vi "Check Slave Name.vi"(8 "error in (no error)":errorcluster, 9 "Prepend in":bool, 10 "Slave Name In":string, 11 "Item Ref in":T1 format="%.0x") -> (0 "error out":errorcluster, 1 "Prepend out":bool, 2 "Available?":bool, 3 "Item Ref out":T1 format="%.0x", 4 "Slave Name":string)   [LabVIEW 2020, in "SEECD System Explorer.lvlib"]
uses:
  SEECD System Explorer.lvlib
  <vilib>/NI VeriStand/Custom Device API/Custom Device API.lvlib
  <vilib>/NI VeriStand/Custom Device API/Custom Device Item Ref.ctl
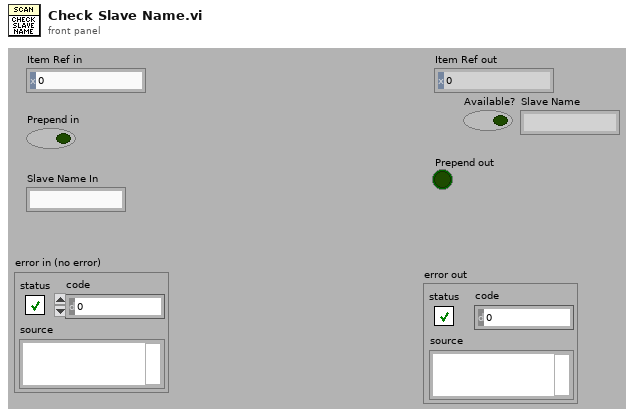
[diagram p1: front panel]
types:
  T1 = typedef "Custom Device API.lvlib/Custom Device Item Ref.ctl" = u64
  T2 = typedef "Custom Device API.lvlib/Custom Device Item Info.ctl" = cluster{"Name":string, "Is Channel":bool, "GUID":string, "Is Waveform":bool}
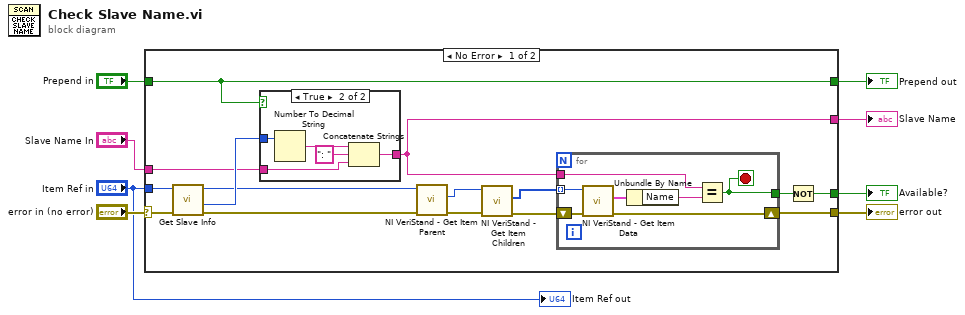
[diagram p0: block diagram]
diagram:
  n1 = case shown="No Error" "error in (no error)" {
    selector: "error in (no error)" -> [w15 w38]
    tunnel: [w20 w38] -> w7
    tunnel: "Item Ref in" -> [w16 _]
    tunnel: "Prepend in" -> [w14 w37]
    tunnel: [w14 w37] -> w5
    tunnel: [w19 _] -> w4
    tunnel: [w10 _] -> w2
    tunnel: "Slave Name In" -> [w9 _]
    frame No Error {
      n2 = call "Get Slave Info.vi"("error in (no error)"=w15, "Item Ref in"=w16) -> ("error out"=w11:errorcluster, "Slave #"=w13:u16, "Item Ref out"=w12:T1)  [unwired: 4 in, 3 out]
      n3 = case shown="True" w14 {
        tunnel: [w24 w29] -> w10
        tunnel: w9 -> [w24 w28]
        tunnel: w13 -> [_ w27]
        frame False {
        }
        frame True {
          n4 = Number To Decimal String(number=w27) -> (decimal integer string=w26:string)  [unwired: 1 in]
          n5 = Concatenate Strings(w26, ": " ("string"), w28) -> (w29:string)
        }
      }
      n6 = call <vilib>:"NI VeriStand - Get Item Parent.vi"("error in (no error)"=w11, "Item Ref in"=w12) -> ("error out"=w18:errorcluster, "Parent Ref"=w17:T1)  [unwired: 6 in, 2 out]
      n7 = call <vilib>:"NI VeriStand - Get Item Children.vi"("error in (no error)"=w18, "Item Ref in"=w17) -> ("error out"=w23:errorcluster, "Child Refs"=w22:T1[])  [unwired: 6 in, 2 out]
      n8 = for {
        tunnel: w22 -> [w34] mode=indexing
        shift-right: [w31] -> w20
        shift-left: w23 -> [w33]
        tunnel: [w36] -> w21
        tunnel: w10 -> [w30]
        stop <- w36 stop-if-true
        n9 = call <vilib>:"NI VeriStand - Get Item Data.vi"("error in (no error)"=w33, "Item Ref in"=w34) -> ("error out"=w31:errorcluster, "Item Info"=w35:T2)  [unwired: 8 out]
        n10 = Unbundle By Name(w35) -> ("Name"=w32:string)
        n11 = Equal?(x=w30, y=w32) -> (x = y?=w36:bool)
      }
      n12 = Not(x=w21) -> (.not. x?=w19:bool)
    }
    frame Error {
    }
  }
  "error out" <- w7
  "Available?" <- w4
  "Prepend out" <- w5
  "Slave Name" <- w2
  "Item Ref out" <- "Item Ref in"
